vi "exit-tasks.vi"(2 "Message Queues out":T1, 4 "test mode":T2(ring)) -> (10 "error out":errorcluster)   [LabVIEW 2015]
uses:
  support/Message Queue/All Message Queues.ctl
  support/Message Queue/Message Cluster.ctl
  support/Message Queue/Enqueue Message (Single).vi
  support/Message Queue/Enqueue Message (Array).vi
  support/Message Queue/Message Queue.lvlib
panel:
  in  "error in (no error)":errorcluster
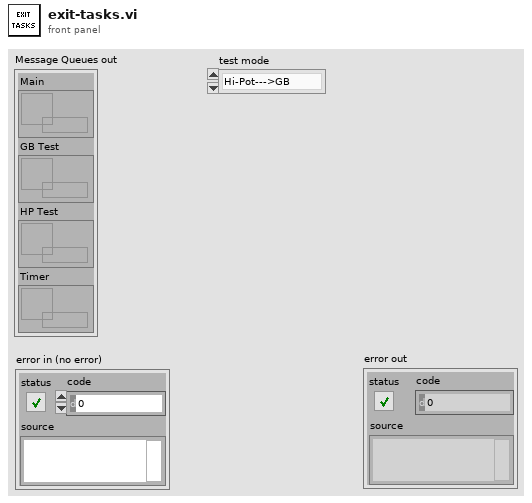
[diagram p1: front panel]
types:
  T1 = typedef "Message Queue.lvlib/All Message Queues.ctl" = cluster{"Main":refnum<queue>, "GB Test":refnum<queue>, "HP Test":refnum<queue>, "Timer":refnum<queue>}
  T2 = enum16{"Hi-Pot--->GB", "GB--->Hi-Pot", "Hi-Pot only", "GB only"}
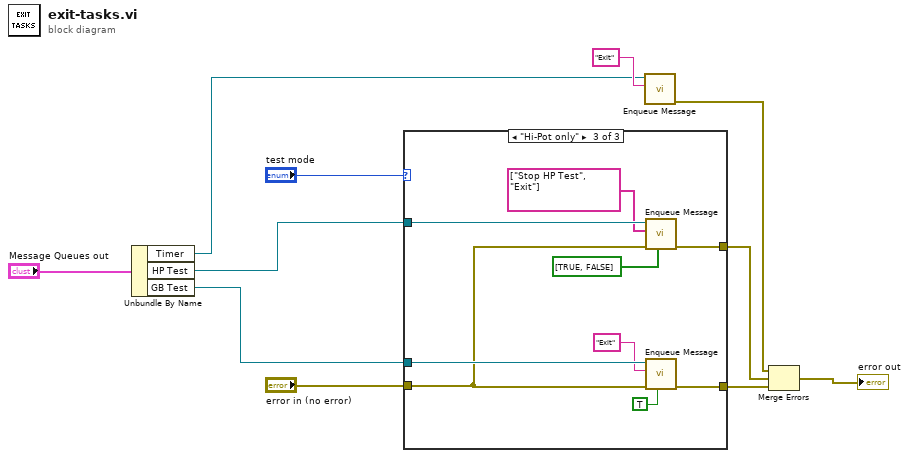
[diagram p0: block diagram]
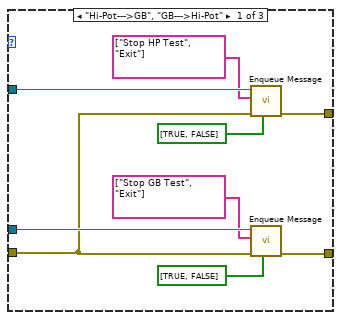
[diagram p2: hidden frame]
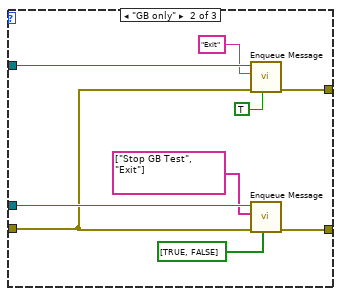
[diagram p3: hidden frame]
diagram:
  n1 = Unbundle By Name("Message Queues out") -> ("Timer"=w2:refnum<queue>, "HP Test"=w4:refnum<queue>, "GB Test"=w3:refnum<queue>)
  n2 = case shown="\"Hi-Pot only\"" "test mode" {
    tunnel: w3 -> [w18 w28 w36]
    tunnel: w4 -> [w17 w27 w37]
    tunnel: [w16 w24 w34] -> w10
    tunnel: [w15 w23 w33] -> w9
    tunnel: "error in (no error)" -> [w12 w21 w30]
    frame "Hi-Pot--->GB", "GB--->Hi-Pot" {
      n3 = call-poly "Enqueue Message.vi"("Priority Message? Array"=bool[] [TRUE, FALSE], "error in (no error)"=w12, "Message Array"=string[] ["Stop HP Test", "Exit"], "Message Queue"=w17) -> ("error out"=w16:errorcluster)  [unwired: 6 in, 1 out]
      n4 = call-poly "Enqueue Message.vi"("Priority Message? Array"=bool[] [TRUE, FALSE], "error in (no error)"=w12, "Message Array"=string[] ["Stop GB Test", "Exit"], "Message Queue"=w18) -> ("error out"=w15:errorcluster)  [unwired: 6 in, 1 out]
    }
    frame "GB only" {
      n5 = call-poly "Enqueue Message.vi"("Priority Message? (F)"=TRUE, "error in (no error)"=w21, "Message"="Exit", "Message Queue"=w27) -> ("error out"=w24:errorcluster)  [unwired: 6 in, 1 out]
      n6 = call-poly "Enqueue Message.vi"("Priority Message? Array"=bool[] [TRUE, FALSE], "error in (no error)"=w21, "Message Array"=string[] ["Stop GB Test", "Exit"], "Message Queue"=w28) -> ("error out"=w23:errorcluster)  [unwired: 6 in, 1 out]
    }
    frame "Hi-Pot only" {
      n7 = call-poly "Enqueue Message.vi"("Priority Message? Array"=bool[] [TRUE, FALSE], "error in (no error)"=w30, "Message Array"=string[] ["Stop HP Test", "Exit"], "Message Queue"=w37) -> ("error out"=w34:errorcluster)  [unwired: 6 in, 1 out]
      n8 = call-poly "Enqueue Message.vi"("Priority Message? (F)"=TRUE, "error in (no error)"=w30, "Message"="Exit", "Message Queue"=w36) -> ("error out"=w33:errorcluster)  [unwired: 6 in, 1 out]
    }
  }
  n9 = call-poly "Enqueue Message.vi"("Message"="Exit", "Message Queue"=w2) -> ("error out"=w1:errorcluster)  [unwired: 8 in, 1 out]
  n10 = Merge Errors(w1, w10, w9) -> (→"error out":errorcluster)
